vi "LP Motor Thread.vi"(11 "VISA resource name":refnum<visa-resource-name>="ASRL3::INSTR") -> ()   [LabVIEW 2015]
uses:
  MCode_LV_86/MDrive Mode.ctl
  MCode_LV_86/Set Parameter.ctl
  Stream/LP Globals.vi
  Stream/Controls/LP Motor CMD.ctl
  Stream/Controls/LP Motor Instruction.ctl
  Controls/LP Axis Enum Typedef.ctl
  Controls/LP Absolute Position Typedef.ctl
  Stream/Controls/Motor Loop Mode Typedef.ctl
  Controls/LP Motor Thread Data.ctl
  Stream/Controls/RT Streamer State.ctl
  Stream/Controls/RT Streamer Queue element.ctl
  Stream/RT Controls/RT Streamer Ack element.ctl
  MCode_LV_86/Get Parameter.ctl
  Stream/Controls/LP System State Typedef.ctl
  <vilib>/platform/TimedLoop/XDataNode/XDataNode.xnode
  <vilib>/Platform/TimedLoop/XDataNode/nitl_modes.ctl
  <vilib>/Platform/TimedLoop/XDataNode/XDNodeRunTimeDep.lvlib
  <vilib>/Platform/TimedLoop/XDataNode/wakeup.ctl
  <vilib>/Platform/TimedLoop/XDataNode/timing_clust.ctl
  Stream/Controls/LP Motor Pos And State.ctl
panel:
  out "MovedY":bool
  out "MovedR":bool
  out "MovedP":bool
  out "last error":errorcluster
  out "semaphore":T1
  out "MotorLoopMode":T2=enum."Open Loop"
  out "Working Velocity":string="10000"
  out "Hold Current":string="5"
  out "Run Current":string="50"
  out "Decel Setpoint":string="60000"
  out "Velocity":i32=10000
  out "Pitch Gain":i32=3000
  out "Roll Gain":i32=-3000
  out "RT Loop Error":errorcluster
  out "Closed Loope Cycle Time":u32
  out "open Loope Cycle Time":u32
  out "output cluster":T3
  out "MotPosition":T4
  out "CMD":T5
  out "error out":errorcluster
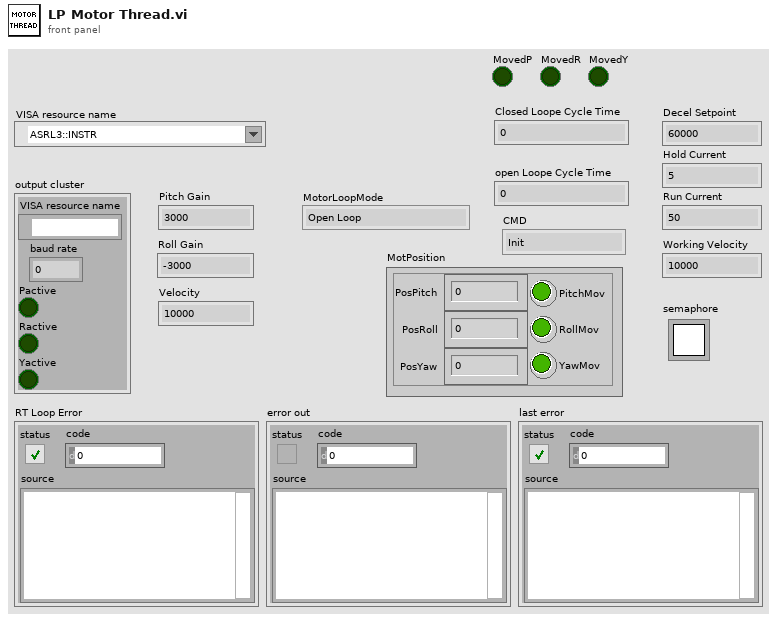
[diagram p1: front panel]
types:
  T1 = typedef "Semaphore RefNum" = refnum<k1>
  T2 = typedef "Motor Loop Mode Typedef.ctl" = enum16{"NotActive", "Open Loop", "Closed Loop", "ClosedOnce"}
  T3 = typedef "LP Motor Thread Data.ctl" = cluster{"VISA resource name":refnum<visa-resource-name>, "baud rate":u32, "Pactive":bool, "Ractive":bool, "Yactive":bool}
  T4 = typedef "LP Motor Pos And State.ctl" = cluster{"PosPitch":dbl, "PosRoll":dbl, "PosYaw":dbl, "PitchMov":bool, "RollMov":bool, "YawMov":bool}
  T5 = typedef "LP Motor CMD.ctl" = enum16{"Init", "SetAccelaration", "SetMaxVelocity", "Idle", "ClosedLoopRun", "MoveAbsolute", "MoveRelative", "MoveSRelative", "MoveSAbsolute", "StopMotors", "EnabeMotors", "SetZero", "StopMotion", "SetLoop", "FindHome", "MotorsGoToLimits", "ErrorHandling", "CloseMotor"}
  T6 = typedef "RT Streamer Ack element.ctl" = cluster{"Data":variant, "CMD":string, "error":errorcluster}
  T7 = typedef "LP System State Typedef.ctl" = cluster{"AutoLevel":bool, "MotorsEngaged":bool, "IMUok":bool}
  T8 = typedef "LP Motor Instruction.ctl" = cluster{"CMD":T5, "Data":variant}
  T9 = typedef "XDNodeRunTimeDep.lvlib/timing_clust.ctl" = cluster{"Expected End [f-1]":u64, "Actual End [f-1]":u64, "Finished Late? [f-1]":bool, "Expected End [i-1]":u64, "Actual End [i-1]":u64, "Finished Late? [i-1]":bool, "Expected Start [i]":u64, "Actual Start [i]":u64, "Expected Start [f]":u64, "Actual Start [f]":u64, "Source Name":string, "Structure Name":string, "Period":i64, "Deadline":i64, "Offset":i64, "Start":i64, "Priority":i32, "Timeout":i32, "Mode":T10, "Wakeup Reason":T11, "Error":errorcluster, "Source Type":string, "Secondary Source Type":string, "Global End Time":u64, "Global Start Time":u64, "Frame Duration":u64, "Iteration Duration":u64, "Assigned CPU":i32, "I/O Scan Engine Mode":u32}
  T10 = typedef "XDNodeRunTimeDep.lvlib/nitl_modes.ctl" = enum32{"No Change", "Process missed periods, maintain original phase", "Discard missed periods, maintain original phase", "Process missed periods, ignore original phase", "Discard missed periods, ignore original phase"}
  T11 = typedef "XDNodeRunTimeDep.lvlib/wakeup.ctl" = enum32{"Normal", "Aborted", "Asynchronous wakeup", "Timing source error", "Timed loop error", "Timeout"}
  T12 = typedef "LP Absolute Position Typedef.ctl" = cluster{"Axis":T13, "Position":dbl}
  T13 = typedef "LP Axis Enum Typedef.ctl" = enum16{"Pitch", "Roll", "Yaw"}
  T14 = typedef "Set Parameter.ctl" = enum16{"Acceleration (A)", "Baud Rate (BD)", "Counter 1 (C1)", "Counter 2 (C2)", "Control C Software Reset (CE)", "Check Sum Enable (CK)", "Clock Mode (CM)", "Clock Mode Ratio (CR)", "Clock Mode Out Step Width (CW)", "Deceleration (D)", "Digital Filtering, Input 1 (D1)", "Digital Filtering, Input 2 (D2)", "Digital Filtering, Input 3 (D3)", "Digital Filtering, Input 4 (D4)", "Digital Filtering, Input 5 (D5)", "Digital Filtering, Input 9 (D9)", "Digital Filtering, Input 10 (D10)", "Digital Filtering, Input 11 (D11)", "Digital Filtering, Input 12 (D12)", "Deadband (DB)", "Decrement Variable (DC)", "Enable/Disable Drive (DE)", "Device Name (DN)", "End Program Execution (E)", "Encoder Function Enable (EE)", "Encoder Lines (EL)", "Echo Mode (EM)", "Error Clear (ER)", "Escape (ES)", "Execute Program at Address (EX)", "Factory Default (FD)", "Hold (H)", "Hold Current (HC)", "Hold Current Encoder Index (HI)", "Home to Home Switch (HM)", "Home to Delay Time (HT)", "Increment Variable (IC)", "Initialize Parameters to NVM (IP)", "Input into Variable (IV)", "Jog Enable (JE)", "Limit Stop Mode (LM)", "Move Absolute (MA)", "Move Relative (MR)", "MicroStepping Select (MS)", "Motor Settling Delay Time (MT)", "Output 1 (O1)", "Output 2 (O2)", "Output 3 (O3)", "Output 4 (O4)", "Output 9 (O9)", "Output 10 (O10)", "Output 11 (O11)", "Output 12 (O12)", "Output High Byte (9-12) (OH)", "Output Low Byte (1-4) (OL)", "Output Total (1-4 and 9-12) (OT)", "Position (P)", "Position Maintenance (PM)", "Party Mode (PY)", "Register 1 (R1)", "Register 2 (R2)", "Register 3 (R3)", "Register 4 (R4)", "Run Current (RC)", "Stall Factor (SF)", "Slew (SL)", "Stall Mode Set (SM)", "Upgrade Firmware (UG)", "Velocity Initial (VI)", "Velocity Maximum (VM)", "Set Input #1 as Home (S1)", "Save (S)", "Save DN+PY (NameS)", "Active Party Mode (0x0A)", "Set Input #1 (S1) as Limit- Active Floating", "Set Input #2 (S2) as Limit+ Active Floating", "Set Input #1 as Home (S1) Active Floating", "Set Input #1 as Home (S2) Active Floating", "Set Input #1 (S1) as Limit+ Active Floating", "Set Input #2 (S2) as Limit- Active Floating", "Hybrid Mode (AS)"}
  T15 = typedef "RT Streamer Queue element.ctl" = cluster{"CMD":T16, "Data":variant}
  T16 = typedef "RT Streamer State.ctl" = enum16{"Init", "Idle", "Stream", "Listen", "SetRefrashRate", "SendCmdAck", "SendCmdDone", "SendSysState", "StartRecord", "Error"}
  T17 = typedef "MDrive Mode.ctl" = enum16{"Normal Mode", "Party Mode"}
  T18 = typedef "Get Parameter.ctl" = enum16{"Acceleration (A)", "Baud Rate (BD)", "Busy Flag (BY)", "Counter 1 (C1)", "Counter 2 (C2)", "Check Sum Enable (CK)", "Clock Mode (CM)", "Clock Mode Ratio (CR)", "Clock Mode Out Step Width (CW)", "Deceleration (D)", "Digital Filtering, Input 1 (D1)", "Digital Filtering, Input 2 (D2)", "Digital Filtering, Input 3 (D3)", "Digital Filtering, Input 4 (D4)", "Digital Filtering, Input 5 (D5)", "Digital Filtering, Input 9 (D9)", "Digital Filtering, Input 10 (D10)", "Digital Filtering, Input 11 (D11)", "Digital Filtering, Input 12 (D12)", "Deadband (DB)", "Enable/Disable Drive (DE)", "Device Name (DN)", "End Program Execution (E)", "Encoder Function Enable (EE)", "Encoder Lines (EL)", "Error Flag (EF)", "Error Variable (ER)", "Echo Mode (EM)", "Escape (ES)", "Execute Program at Address (EX)", "Hold Current (HC)", "Hold Current Delay Time (HI)", "Input 1 (I1)", "Input 2 (I2)", "Input 3 (I3)", "Input 4 (I4)", "Input 5 Analog (I5)", "Input 6 Encoder Index (I6)", "Input 9 (I9)", "Input 10 (I10)", "Input 11 (I11)", "Input 12 (I12)", "Input Low Byte (1-4) (IL)", "Input High Byte (9-12) (IH)", "Inputs Total (1-4,9-12) (IN)", "Internal Temperature (IT)", "Jog Enable (JE)", "Limit Stop Mode (LM)", "MicroStepping Select (MS)", "Motor Settling Delay Time (MT)", "Moving Flag (MV)", "Output 1 (O1)", "Output 2 (O2)", "Output 3 (O3)", "Output 4 (O4)", "Output 9 (O9)", "Output 10 (O10)", "Output 11 (O11)", "Output 12 (O12)", "Output High Byte (9-12) (OH)", "Output Low Byte (1-4) (OL)", "Output Total (1-4 and 9-12) (OT)", "Position (P)", "Position Captured at Trip (PC)", "Position Maintenance (PM)", "Part Number (PN)", "Party Mode (PY)", "Register 1 (R1)", "Register 2 (R2)", "Register 3 (R3)", "Register 4 (R4)", "Run Current (RC)", "Serial Number (SN)", "Stall Flag (ST)", "Stall Factor (SF)", "Stall Mode Set (SM)", "User Variables (UV)", "Velocity (V)", "Velocity Changing Flag (VC)", "Velocity Initial (VI)", "Version, Firmware (VR)", "Velocity Maximum (VM)", "Read Input1", "Read Input2"}
  T19 = cluster{dbl, i32, dbl, "MovingFlag":bool, "MovingFlag":bool, "MovingFlag":bool}
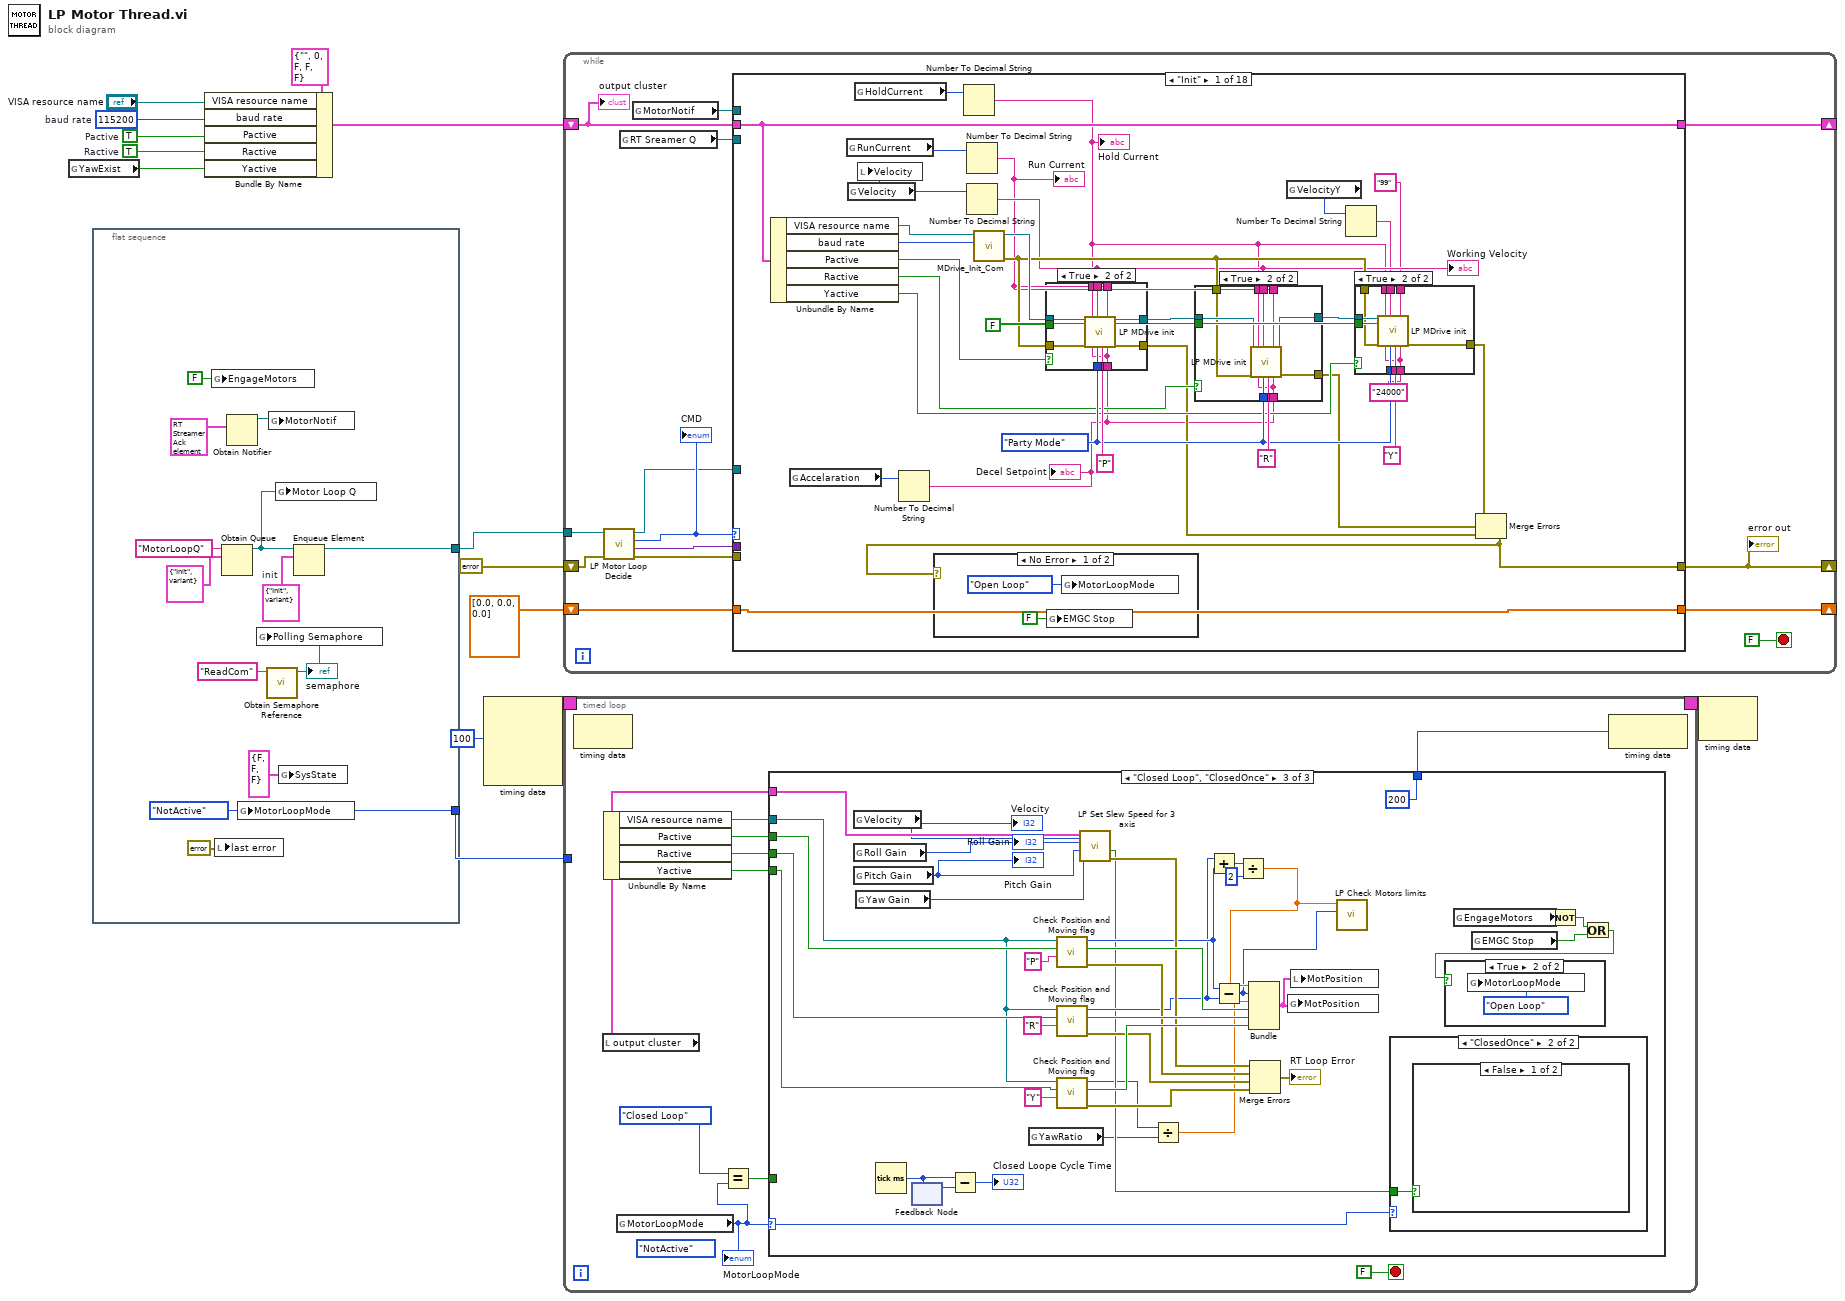
[diagram p0: block diagram]
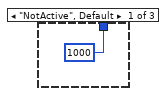
[diagram p2: hidden frame]
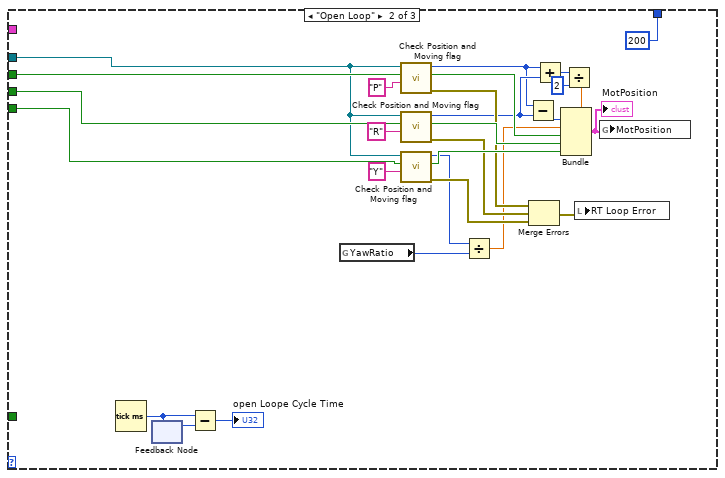
[diagram p3: hidden frame]
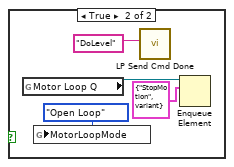
[diagram p6: hidden frame]
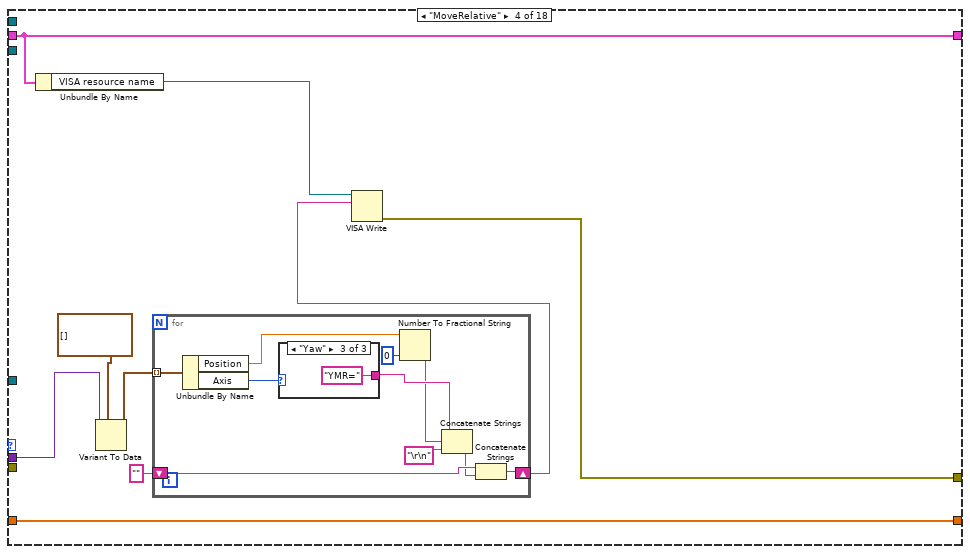
[diagram p13: hidden frame]
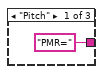
[diagram p14: hidden frame]
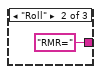
[diagram p15: hidden frame]
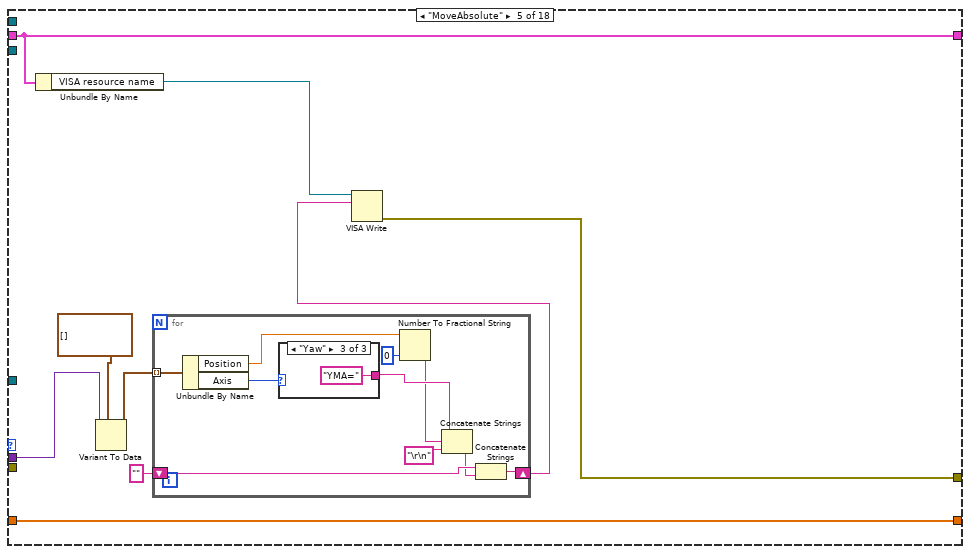
[diagram p16: hidden frame]
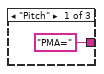
[diagram p17: hidden frame]
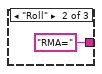
[diagram p18: hidden frame]
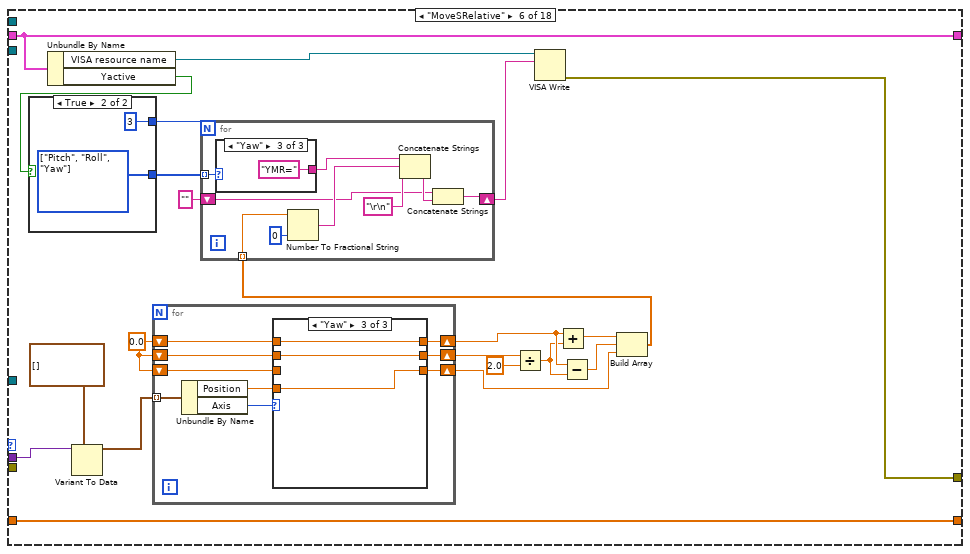
[diagram p19: hidden frame]
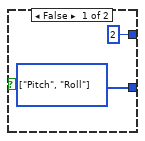
[diagram p20: hidden frame]
diagram:
  w7 = TRUE  # Ractive
  w8 = TRUE  # Pactive
  w12 = u32 115200  # baud rate
  n1 = global read "LP Globals.vi" "YawExist"() -> (w4:bool)
  n2 = flat-sequence {
    tunnel: [w23] -> w10
    tunnel: [w25] -> w9
    frame #0 {
      w22 = T8 {"CMD"=enum."Init", "Data"=variant}  # init
      w25 = Motor_Loop_Mode_Typedef."NotActive" ("MotorLoopMode")
      n3 = global write "LP Globals.vi" "EngageMotors"(FALSE ("EngageMotors")) -> ()
      n4 = local write "last error"(errorcluster {"status"=FALSE, "code"=0, "source"=""} ("last error")) -> ()
      n5 = Obtain Queue(name (unnamed)="MotorLoopQ", element data type=T8 {"CMD"=enum."Init", "Data"=variant} ("Motor Instruction")) -> (queue out=w24:refnum<queue>)  [unwired: 3 in, 2 out]
      n6 = Obtain Notifier(notification data type=T6 {"Data"=variant, "CMD"="", "error"={"status"=FALSE, "code"=0, "source"=""}} ("Cluster")) -> (notifier out=w16:refnum<notifier>)  [unwired: 3 in, 2 out]
      n7 = global write "LP Globals.vi" "MotorLoopMode"(w25) -> ()
      n8 = call <vilib>:"Obtain Semaphore Reference.vi"("name (unnamed)"="ReadCom") -> ("semaphore"=w20:T1)  [unwired: 4 in, 2 out]
      "semaphore" <- w20
      n9 = global write "LP Globals.vi" "Polling Semaphore"(w20) -> ()
      n10 = global write "LP Globals.vi" "MotorNotif"(w16) -> ()
      n11 = global write "LP Globals.vi" "Motor Loop Q"(w24) -> ()
      n12 = global write "LP Globals.vi" "SysState"(T7 {"AutoLevel"=FALSE, "MotorsEngaged"=FALSE, "IMUok"=FALSE} ("SysState")) -> ()
      n13 = Enqueue Element(queue=w24, element=w22) -> (queue out=w23:refnum<queue>)  [unwired: 2 in, 2 out]
    }
  }
  n14 = Bundle By Name(cluster=T3 {"VISA resource name"="", "baud rate"=0, "Pactive"=FALSE, "Ractive"=FALSE, "Yactive"=FALSE} ("output cluster"), "VISA resource name"="VISA resource name", "baud rate"=w12, "Pactive"=w8, "Ractive"=w7, "Yactive"=w4) -> (w11:T3)
  n15 = node-c288(i64 100 ("Period")) -> (w3:T9)  [unwired: 3 in]
  n16 = while {
    tunnel: w10 -> [w40]
    shift-right: [w36] -> _
    shift-left: errorcluster {"status"=FALSE, "code"=0, "source"=""} ("error out") -> [w38]
    shift-right: [w37] -> _
    shift-left: w11 -> [w32]
    shift-right: [w30] -> _
    shift-left: dbl[] [0.0, 0.0, 0.0] -> [w31]
    stop <- FALSE stop-if-true
    n17 = call "LP Motor Loop Decide.vi"("error in (no error)"=w38, "Queue in"=w40) -> ("error out"=w39:errorcluster, "Data"=w35:variant, "CMD"=w34:T5, "queue out"=w33:refnum<queue>)  [unwired: 6 in]
    "CMD" <- w34
    n18 = global read "LP Globals.vi" "RT Sreamer Q"() -> (w29:refnum<queue>)
    n19 = global read "LP Globals.vi" "MotorNotif"() -> (w28:refnum<notifier>)
    n20 = case shown="\"Init\"" w34 {
      tunnel: w35 -> [_ _ _ w124 w146 w180 _ w238 w292 w307 _ w362 _ w462 _ _ _ _]
      tunnel: w39 -> [_ w113 w114 _ _ _ _ _ _ _ _ _ _ _ _ _ w535 w540]
      tunnel: [w55 w113 w114 w118 w140 w176 w217 w234 w286 w305 w328 w350 w427 w461 w476 w507 _ w540] -> w36
      tunnel: w32 -> [w71 w112 w116 w125 w147 w181 w218 w239 w294 w309 w334 w371 w443 w466 w482 w511 w536 w539]
      tunnel: [w71 w112 w116 w125 w147 w181 w218 w239 w294 w309 w334 w371 w443 w466 w482 w511 w536 w539] -> w37
      tunnel: w33 -> [_ _ _ _ _ _ _ _ _ _ _ _ _ w460 _ _ _ _]
      tunnel: w31 -> [w54 w111 w115 w117 w139 w164 w216 w225 w281 w302 w323 w361 w433 w459 w471 w499 w533 w537]
      tunnel: [w54 w111 w115 w117 w139 w164 w216 w224 w281 w302 w323 w361 w433 w459 w471 w499 w533 w537] -> w30
      tunnel: w29 -> [_ _ _ _ _ _ _ _ _ _ _ _ w432 _ _ _ _ _]
      tunnel: w28 -> [_ _ _ _ _ _ _ _ _ _ _ _ w426 _ _ _ _ _]
      frame "Init" {
        w63 = FALSE ("Factory Default")
        w65 = MDrive_Mode."Party Mode" ("Mdrive Mode")
        n21 = Unbundle By Name(w71) -> ("VISA resource name"=w73:refnum<visa-resource-name>, "baud rate"=w72:u32, "Pactive"=w62:bool, "Ractive"=w61:bool, "Yactive"=w60:bool)
        n22 = global read "LP Globals.vi" "Accelaration"() -> (w52:i32)
        n23 = global read "LP Globals.vi" "RunCurrent"() -> (w48:i32)
        n24 = global read "LP Globals.vi" "Velocity"() -> (w46:i32)
        n25 = global read "LP Globals.vi" "HoldCurrent"() -> (w50:i32)
        n26 = local write "Velocity"(w46) -> ()
        n27 = Number To Decimal String(number=w52) -> (decimal integer string=w51:string)  [unwired: 1 in]
        "Decel Setpoint" <- w51
        n28 = Number To Decimal String(number=w50) -> (decimal integer string=w49:string)  [unwired: 1 in]
        "Hold Current" <- w49
        n29 = Number To Decimal String(number=w48) -> (decimal integer string=w47:string)  [unwired: 1 in]
        "Run Current" <- w47
        n30 = Number To Decimal String(number=w46) -> (decimal integer string=w53:string)  [unwired: 1 in]
        "Working Velocity" <- w53
        n31 = call "MDrive_Init_Com.vi"("baud rate"=w72, "VISA resource name"=w73) -> ("error out"=w56:errorcluster, "VISA resource name out"=w70:refnum<visa-resource-name>)  [unwired: 8 in]
        n32 = case shown="True" w62 {
          tunnel: w70 -> [w97 w108]
          tunnel: [w97 w107] -> w69
          tunnel: [w96 w99] -> w57
          tunnel: "P" ("Device Name") -> [_ w106]
          tunnel: w65 -> [_ w105]
          tunnel: w51 -> [_ w104]
          tunnel: w47 -> [_ w103]
          tunnel: w49 -> [_ w102]
          tunnel: w53 -> [_ w101]
          tunnel: w63 -> [_ w100]
          tunnel: w56 -> [w96 w98]
          frame False {
          }
          frame True {
            n33 = call "LP MDrive init.vi"("VISA IN"=w108, "Factory Default"=w100, "error in"=w98, "Hold Current"=w102, "Accel Setpoint"=w104, "Working Velocity"=w101, "Mdrive Mode"=w105, "Device Name"=w106, "Run Current"=w103, "Decel Setpoint"=w104) -> ("VISA OUT"=w107:refnum<visa-resource-name>, "error out"=w99:errorcluster)  [unwired: 8 in]
          }
        }
        n34 = case shown="True" w61 {
          tunnel: w69 -> [w84 w95]
          tunnel: "R" ("Device Name") -> [_ w94]
          tunnel: [_ w93] -> w58
          tunnel: [w84 w92] -> w66
          tunnel: w65 -> [_ w91]
          tunnel: w51 -> [_ w90]
          tunnel: w47 -> [_ w89]
          tunnel: w49 -> [_ w88]
          tunnel: w53 -> [_ w87]
          tunnel: w63 -> [_ w86]
          tunnel: w56 -> [_ w85]
          frame False {
          }
          frame True {
            n35 = call "LP MDrive init.vi"("VISA IN"=w95, "Factory Default"=w86, "error in"=w85, "Hold Current"=w88, "Accel Setpoint"=w90, "Working Velocity"=w87, "Mdrive Mode"=w91, "Device Name"=w94, "Run Current"=w89, "Decel Setpoint"=w90) -> ("VISA OUT"=w92:refnum<visa-resource-name>, "error out"=w93:errorcluster)  [unwired: 8 in]
          }
        }
        n36 = global read "LP Globals.vi" "VelocityY"() -> (w43:i32)
        n37 = Number To Decimal String(number=w43) -> (decimal integer string=w45:string)  [unwired: 1 in]
        n38 = case shown="True" w60 {
          tunnel: w66 -> [_ w83]
          tunnel: w65 -> [_ w82]
          tunnel: "Y" ("Device Name") -> [_ w81]
          tunnel: "24000" -> [_ w80]
          tunnel: "99" ("decimal integer string") -> [_ w79]
          tunnel: w49 -> [_ w78]
          tunnel: [_ w77] -> w59
          tunnel: w63 -> [_ w76]
          tunnel: w56 -> [_ w75]
          tunnel: w45 -> [_ w74]
          frame False {
          }
          frame True {
            n39 = call "LP MDrive init.vi"("VISA IN"=w83, "Factory Default"=w76, "error in"=w75, "Hold Current"=w78, "Accel Setpoint"=w80, "Working Velocity"=w74, "Mdrive Mode"=w82, "Device Name"=w81, "Run Current"=w79, "Decel Setpoint"=w80) -> ("error out"=w77:errorcluster)  [unwired: 8 in, 1 out]
          }
        }
        n40 = Merge Errors(w59, w58, w57) -> (w55:errorcluster)
        n41 = case shown="No Error" w55 {
          frame No Error {
            n42 = global write "LP Globals.vi" "EMGC Stop"(FALSE ("EMGC Stop")) -> ()
            n43 = global write "LP Globals.vi" "MotorLoopMode"(Motor_Loop_Mode_Typedef."Open Loop" ("MotorLoopMode")) -> ()
          }
          frame Error {
          }
        }
      }
      frame "Idle" {
      }
      frame "ClosedLoopRun" {
      }
      frame "MoveRelative" {
        n44 = Unbundle By Name(w125) -> ("VISA resource name"=w119:refnum<visa-resource-name>)
        n45 = Variant To Data(type=T12[] [], Variant=w124) -> (data=w123:T12[])  [unwired: 1 in, 1 out]
        n46 = for {
          tunnel: w123 -> [w135] mode=indexing
          shift-right: [w126] -> w120
          shift-left: "" -> [w128]
          n47 = Unbundle By Name(w135) -> ("Position"=w133:dbl, "Axis"=w134:T13)
          n48 = case shown="\"Yaw\"" w134 {
            tunnel: ["PMR=" "RMR=" "YMR="] -> w131
            frame "Pitch" {
            }
            frame "Roll" {
            }
            frame "Yaw" {
            }
          }
          n49 = Number To Fractional String(number=w133, precision (6)=i16 0) -> (F-format string=w130:string)  [unwired: 2 in]
          n50 = Concatenate Strings(w131, w130, "\r\n") -> (w127:string)
          n51 = Concatenate Strings(w128, w127) -> (w126:string)
        }
        n52 = VISA Write(VISA resource name=w119, write buffer=w120) -> (error out=w118:errorcluster)  [unwired: 1 in, 2 out]
      }
      frame "MoveAbsolute" {
        n53 = Unbundle By Name(w147) -> ("VISA resource name"=w141:refnum<visa-resource-name>)
        n54 = Variant To Data(type=T12[] [], Variant=w146) -> (data=w145:T12[])  [unwired: 1 in, 1 out]
        n55 = for {
          tunnel: w145 -> [w157] mode=indexing
          shift-right: [w148] -> w142
          shift-left: "" -> [w150]
          n56 = Unbundle By Name(w157) -> ("Position"=w155:dbl, "Axis"=w156:T13)
          n57 = case shown="\"Yaw\"" w156 {
            tunnel: ["PMA=" "RMA=" "YMA="] -> w153
            frame "Pitch" {
            }
            frame "Roll" {
            }
            frame "Yaw" {
            }
          }
          n58 = Number To Fractional String(number=w155, precision (6)=i16 0) -> (F-format string=w152:string)  [unwired: 2 in]
          n59 = Concatenate Strings(w153, w152, "\r\n") -> (w149:string)
          n60 = Concatenate Strings(w150, w149) -> (w148:string)
        }
        n61 = VISA Write(VISA resource name=w141, write buffer=w142) -> (error out=w140:errorcluster)  [unwired: 1 in, 2 out]
      }
      frame "MoveSRelative" {
        w175 = 0.0 ("Position")
        n62 = Unbundle By Name(w181) -> ("VISA resource name"=w177:refnum<visa-resource-name>, "Yactive"=w161:bool)
        n63 = case shown="True" w161 {
          tunnel: [w183 w185] -> w169
          tunnel: [2 3] -> w162
          frame False {
            w183 = T13[] [enum."Pitch", enum."Roll"] items=["Pitch", "Roll", "Yaw"]
          }
          frame True {
            w185 = T13[] [enum."Pitch", enum."Roll", enum."Yaw"] items=["Pitch", "Roll", "Yaw"]
          }
        }
        n64 = Variant To Data(type=T12[] [], Variant=w180) -> (data=w179:T12[])  [unwired: 1 in, 1 out]
        n65 = for {
          tunnel: w179 -> [w206] mode=indexing
          shift-right: [w202] -> w174
          shift-left: w175 -> [w200]
          shift-right: [w204] -> w172
          shift-left: w175 -> [w198]
          shift-right: [w201] -> w163
          shift-left: w175 -> [w199]
          n66 = Unbundle By Name(w206) -> ("Position"=w203:dbl, "Axis"=w205:T13)
          n67 = case shown="\"Yaw\"" w205 {
            tunnel: [w207 w212 w215] -> w204
            tunnel: w203 -> [w207 w210 w213]
            tunnel: [w209 w210 w214] -> w202
            tunnel: [w208 w211 w213] -> w201
            tunnel: w200 -> [w209 _ w214]
            tunnel: w199 -> [w208 w211 _]
            tunnel: w198 -> [_ w212 w215]
            frame "Pitch" {
            }
            frame "Roll" {
            }
            frame "Yaw" {
            }
          }
        }
        n68 = Divide(x=w174, y=2.0) -> (x/y=w171:dbl)
        n69 = Add(x=w172, y=w171) -> (x+y=w168:dbl)
        n70 = Subtract(x=w172, y=w171) -> (x-y=w167:dbl)
        n71 = Build Array(w168, w167, w163) -> (w166:dbl[])
        n72 = for {
          N: w162 -> [_]
          shift-right: [w189] -> w165
          shift-left: "" -> [w188]
          tunnel: w169 -> [w187] mode=indexing
          tunnel: w166 -> [w186] mode=indexing
          n73 = case shown="\"Yaw\"" w187 {
            tunnel: ["PMR=" "RMR=" "YMR="] -> w190
            frame "Pitch" {
            }
            frame "Roll" {
            }
            frame "Yaw" {
            }
          }
          n74 = Number To Fractional String(number=w186, precision (6)=i16 0) -> (F-format string=w192:string)  [unwired: 2 in]
          n75 = Concatenate Strings(w190, w192, "\r\n") -> (w194:string)
          n76 = Concatenate Strings(w188, w194) -> (w189:string)
        }
        n77 = VISA Write(VISA resource name=w177, write buffer=w165) -> (error out=w176:errorcluster)  [unwired: 1 in, 2 out]
      }
      frame "MotorsGoToLimits" {
        n78 = call "MotorsGoToLimits.vi"("output cluster"=w218) -> ("error out"=w217:errorcluster)  [unwired: 10 in]
      }
      frame "MoveSAbsolute" {
        n79 = Unbundle By Name(w239) -> ("VISA resource name"=w235:refnum<visa-resource-name>, "Yactive"=w221:bool)
        n80 = case shown="True" w221 {
          tunnel: [w241 w243] -> w230
          tunnel: [2 3] -> w219
          frame False {
            w241 = T13[] [enum."Pitch", enum."Roll"] items=["Pitch", "Roll", "Yaw"]
          }
          frame True {
            w243 = T13[] [enum."Pitch", enum."Roll", enum."Yaw"] items=["Pitch", "Roll", "Yaw"]
          }
        }
        n81 = Variant To Data(type=T12[] [], Variant=w238) -> (data=w237:T12[])  [unwired: 1 in, 1 out]
        n82 = for {
          tunnel: w237 -> [w260] mode=indexing
          shift-right: [w256] -> w224
          shift-left: w225 -> [w257]
          n83 = Unbundle By Name(w260) -> ("Position"=w258:dbl, "Axis"=w259:T13)
          n84 = case shown="\"Pitch\"" w259 {
            tunnel: w258 -> [w262 w268 w274]
            tunnel: w257 -> [w266 w272 w278]
            tunnel: [w264 w270 w276] -> w256
            frame "Pitch" {
              n85 = global read "LP Globals.vi" "PitchRatio"() -> (w263:i32)
              n86 = Multiply(x=w263, y=w262) -> (x*y=w261:dbl)
              n87 = Replace Array Subset(array=w266, new element=w261, index=0) -> (w264:dbl[])
            }
            frame "Roll" {
              n88 = global read "LP Globals.vi" "RollRatio"() -> (w269:i32)
              n89 = Multiply(x=w269, y=w268) -> (x*y=w267:dbl)
              n90 = Replace Array Subset(array=w272, new element=w267, index=1) -> (w270:dbl[])
            }
            frame "Yaw" {
              n91 = global read "LP Globals.vi" "YawRatio"() -> (w273:i32)
              n92 = Multiply(x=w273, y=w274) -> (x*y=w275:dbl)
              n93 = Replace Array Subset(array=w278, new element=w275, index=2) -> (w276:dbl[])
            }
          }
        }
        n94 = Index Array(array=w224) -> (element #1=w223:dbl, element #2=w222:dbl, element #3=w220:dbl)  [unwired: 3 in]
        n95 = Divide(x=w222, y=2.0) -> (x/y=w232:dbl)
        n96 = Add(x=w223, y=w232) -> (x+y=w229:dbl)
        n97 = Subtract(x=w223, y=w232) -> (x-y=w228:dbl)
        n98 = Build Array(w229, w228, w220) -> (w227:dbl[])
        n99 = for {
          N: w219 -> [_]
          shift-right: [w247] -> w226
          shift-left: "" -> [w246]
          tunnel: w230 -> [w245] mode=indexing
          tunnel: w227 -> [w244] mode=indexing
          n100 = case shown="\"Yaw\"" w245 {
            tunnel: ["PMA=" "RMA=" "YMA="] -> w248
            frame "Pitch" {
            }
            frame "Roll" {
            }
            frame "Yaw" {
            }
          }
          n101 = Number To Fractional String(number=w244, precision (6)=i16 0) -> (F-format string=w250:string)  [unwired: 2 in]
          n102 = Concatenate Strings(w248, w250, "\r\n") -> (w252:string)
          n103 = Concatenate Strings(w246, w252) -> (w247:string)
        }
        n104 = VISA Write(VISA resource name=w235, write buffer=w226) -> (error out=w234:errorcluster)  [unwired: 1 in, 2 out]
      }
      frame "SetAccelaration" {
        n105 = Variant To Data(type=T12 {"Axis"=enum."Roll", "Position"=0.0} ("AbsolutePosition"), Variant=w292) -> (data=w290:T12)  [unwired: 1 in, 1 out]
        n106 = Unbundle By Name(w294) -> ("VISA resource name"=w293:refnum<visa-resource-name>)
        n107 = Unbundle By Name(w290) -> ("Position"=w288:dbl, "Axis"=w289:T13)
        n108 = Number To Fractional String(number=w288, precision (6)=i16 0) -> (F-format string=w280:string)  [unwired: 2 in]
        n109 = case shown="\"Yaw\"" w289 {
          tunnel: ["P" "R" "Y"] -> w283
          tunnel: [w296 w298 "24000"] -> w279
          tunnel: w280 -> [w296 w298 _]
          frame "Pitch" {
          }
          frame "Roll" {
          }
          frame "Yaw" {
          }
        }
        n110 = call "MDrive_Set_Parameter.vi"("Device Name"=w283, "Parameter Setpoint"=w279, "Set Parameter"=Set_Parameter."Acceleration (A)", "VISA IN"=w293) -> ("error out"=w287:errorcluster, "VISA OUT"=w285:refnum<visa-resource-name>)  [unwired: 5 in, 1 out]
        n111 = call "MDrive_Set_Parameter.vi"("Device Name"=w283, "error in"=w287, "Parameter Setpoint"=w279, "Set Parameter"=Set_Parameter."Deceleration (D)", "VISA IN"=w285) -> ("error out"=w286:errorcluster)  [unwired: 4 in, 2 out]
      }
      frame "SetMaxVelocity" {
        n112 = Variant To Data(type=T12[] [], Variant=w307) -> (data=w306:T12[])  [unwired: 1 in, 1 out]
        n113 = Unbundle By Name(w309) -> ("VISA resource name"=w308:refnum<visa-resource-name>)
        n114 = for {
          tunnel: w308 -> [w318]
          tunnel: w306 -> [w317] mode=indexing
          shift-right: [w312] -> w305
          shift-left: errorcluster {"status"=FALSE, "code"=0, "source"=""} ("error out") -> [w311]
          n115 = Unbundle By Name(w317) -> ("Position"=w315:dbl, "Axis"=w316:T13)
          n116 = case shown="\"Pitch\"" w316 {
            tunnel: ["P" "R" "Y"] -> w313
            frame "Pitch" {
            }
            frame "Roll" {
            }
            frame "Yaw" {
            }
          }
          n117 = Number To Fractional String(number=w315, precision (6)=i16 0) -> (F-format string=w314:string)  [unwired: 2 in]
          n118 = call "MDrive_Set_Parameter.vi"("Device Name"=w313, "error in"=w311, "Parameter Setpoint"=w314, "Set Parameter"=Set_Parameter."Velocity Maximum (VM)", "VISA IN"=w318) -> ("error out"=w312:errorcluster)  [unwired: 4 in, 2 out]
        }
      }
      frame "StopMotors" {
        (unwired) "0" ("Parameter Setpoint")
        w332 = "\u001b" ("Parameter Setpoint")
        w327 = Set_Parameter."Enable/Disable Drive (DE)" ("Set Parameter")
        n119 = Unbundle By Name(w334) -> ("VISA resource name"=w333:refnum<visa-resource-name>, "Pactive"=w324:bool, "Ractive"=w325:bool, "Yactive"=w326:bool)
        n120 = case shown="True" w326 {
          tunnel: w333 -> [_ w339]
          tunnel: w327 -> [_ w338]
          tunnel: w332 -> [_ w336]
          tunnel: [_ w335] -> w329
          frame False {
          }
          frame True {
            n121 = call "MDrive_Set_Parameter.vi"("Device Name"="Y", "Parameter Setpoint"=w336, "Set Parameter"=w338, "VISA IN"=w339) -> ("error out"=w335:errorcluster)  [unwired: 5 in, 2 out]
          }
        }
        n122 = case shown="True" w325 {
          tunnel: w333 -> [_ w344]
          tunnel: w327 -> [_ w343]
          tunnel: w332 -> [_ w341]
          tunnel: [_ w340] -> w330
          frame False {
          }
          frame True {
            n123 = call "MDrive_Set_Parameter.vi"("Device Name"="R", "Parameter Setpoint"=w341, "Set Parameter"=w343, "VISA IN"=w344) -> ("error out"=w340:errorcluster)  [unwired: 5 in, 2 out]
          }
        }
        n124 = case shown="True" w324 {
          tunnel: w333 -> [_ w349]
          tunnel: w327 -> [_ w348]
          tunnel: w332 -> [_ w346]
          tunnel: [_ w345] -> w331
          frame False {
          }
          frame True {
            n125 = call "MDrive_Set_Parameter.vi"("Device Name"="P", "Parameter Setpoint"=w346, "Set Parameter"=w348, "VISA IN"=w349) -> ("error out"=w345:errorcluster)  [unwired: 5 in, 2 out]
          }
        }
        n126 = Merge Errors(w331, w330, w329) -> (w328:errorcluster)
      }
      frame "EnabeMotors" {
        w359 = u16 2000 ("Timeout")
        w360 = Get_Parameter."Enable/Disable Drive (DE)" ("Get Parameter")
        w369 = Set_Parameter."Enable/Disable Drive (DE)" ("Set Parameter")
        n127 = Unbundle By Name(w371) -> ("VISA resource name"=w370:refnum<visa-resource-name>, "Pactive"=w366:bool, "Ractive"=w365:bool, "Yactive"=w364:bool)
        n128 = Variant To Data(type=TRUE, Variant=w362) -> (data=w351:bool)  [unwired: 1 in, 1 out]
        n129 = case shown="False" w351 {
          tunnel: ["0" ("Parameter Setpoint") "1" ("Parameter Setpoint")] -> w358
          frame False {
          }
          frame True {
          }
        }
        n130 = Decimal String To Number(string=w358) -> (number=w357:i32)  [unwired: 2 in, 1 out]
        n131 = case shown="True" w364 {
          tunnel: w370 -> [_ w404]
          tunnel: w369 -> [_ w403]
          tunnel: w358 -> [_ w402]
          tunnel: [_ w400] -> w367
          tunnel: w360 -> [_ w397]
          tunnel: w359 -> [_ w396]
          tunnel: w357 -> [_ w395]
          frame False {
          }
          frame True {
            w399 = "Y" ("Device Name")
            n132 = call "MDrive_Set_Parameter.vi"("Device Name"=w399, "Parameter Setpoint"=w402, "Set Parameter"=w403, "VISA IN"=w404) -> ("error out"=w401:errorcluster, "VISA OUT"=w398:refnum<visa-resource-name>)  [unwired: 5 in, 1 out]
            n133 = call "Wait For CMD Ack.vi"("Timeout"=w396, "Device Name"=w399, "error in (no error)"=w401, "Get Parameter"=w397, "ExpectedValue"=w395, "VISA Refnum in"=w398) -> ("error out"=w400:errorcluster)  [unwired: 4 in, 1 out]
          }
        }
        n134 = case shown="True" w366 {
          tunnel: w370 -> [_ w424]
          tunnel: w369 -> [_ w423]
          tunnel: w358 -> [_ w422]
          tunnel: [_ w419] -> w356
          tunnel: w360 -> [_ w421]
          tunnel: w359 -> [_ w416]
          tunnel: w357 -> [_ w415]
          frame False {
          }
          frame True {
            w417 = "P" ("Device Name")
            n135 = call "MDrive_Set_Parameter.vi"("Device Name"=w417, "Parameter Setpoint"=w422, "Set Parameter"=w423, "VISA IN"=w424) -> ("error out"=w420:errorcluster, "VISA OUT"=w418:refnum<visa-resource-name>)  [unwired: 5 in, 1 out]
            n136 = call "Wait For CMD Ack.vi"("Timeout"=w416, "Device Name"=w417, "error in (no error)"=w420, "Get Parameter"=w421, "ExpectedValue"=w415, "VISA Refnum in"=w418) -> ("error out"=w419:errorcluster)  [unwired: 4 in, 1 out]
          }
        }
        n137 = case shown="True" w365 {
          tunnel: w370 -> [_ w414]
          tunnel: w369 -> [_ w413]
          tunnel: w358 -> [_ w412]
          tunnel: [_ w410] -> w368
          tunnel: w360 -> [_ w408]
          tunnel: w359 -> [_ w406]
          tunnel: w357 -> [_ w405]
          frame False {
          }
          frame True {
            w409 = "R" ("Device Name")
            n138 = call "MDrive_Set_Parameter.vi"("Device Name"=w409, "Parameter Setpoint"=w412, "Set Parameter"=w413, "VISA IN"=w414) -> ("error out"=w411:errorcluster, "VISA OUT"=w407:refnum<visa-resource-name>)  [unwired: 5 in, 1 out]
            n139 = call "Wait For CMD Ack.vi"("Timeout"=w406, "Device Name"=w409, "error in (no error)"=w411, "Get Parameter"=w408, "ExpectedValue"=w405, "VISA Refnum in"=w407) -> ("error out"=w410:errorcluster)  [unwired: 4 in, 1 out]
          }
        }
        n140 = Merge Errors(w356, w368, w367) -> (w350:errorcluster)
        n141 = case shown="False" w351 {
          tunnel: w350 -> [w388 w391]
          tunnel: [w387 w390] -> w355
          frame False {
            n142 = case shown="No Error" w388 {
              tunnel: [_ w389] -> w387
              frame No Error {
              }
              frame Error {
                n143 = global read "LP Globals.vi" "EngageMotors"() -> (w389:bool)
              }
            }
          }
          frame True {
            n144 = case shown="No Error" w391 {
              tunnel: [TRUE ("EngageMotors") _] -> w390
              frame No Error {
              }
              frame Error {
              }
            }
          }
        }
        n145 = global write "LP Globals.vi" "EngageMotors"(w355) -> ()
        n146 = feedback #1(u8 0) -> (w352:u8)
        n147 = case shown="Error" w350 {
          selector: w350 -> [w372 w376]
          tunnel: [u8 0 w377] -> w353
          tunnel: w352 -> [_ w378]
          tunnel: w351 -> [_ w375]
          frame No Error {
            n148 = call "LP Send Cmd Done.vi"("error in (no error)"=w372, "CMD"="EngageMotor") -> ()  [unwired: 10 in]
          }
          frame Error {
            n149 = case shown="0..3" w378 {
              selector: w378 -> [_ w386]
              tunnel: [_ w385] -> w377
              tunnel: w376 -> [w379 _]
              tunnel: w375 -> [_ w381]
              frame Default {
                n150 = call "LP Send Cmd Done.vi"("error in (no error)"=w379, "CMD"="EngageMotor") -> ()  [unwired: 10 in]
              }
              frame 0..3 {
                n151 = global read "LP Globals.vi" "Motor Loop Q"() -> (w384:refnum<queue>)
                n152 = Increment(x=w386) -> (x+1=w385:u8)
                n153 = Bundle By Name(cluster=T8 {"CMD"=enum."EnabeMotors", "Data"=variant} ("element"), "Data"=w381) -> (w382:T8)
                n154 = Enqueue Element(queue=w384, element=w382) -> ()  [unwired: 2 in, 3 out]
              }
            }
          }
        }
        n155 = feedback-in #1(w353) -> ()
      }
      frame "SetZero" {
        w434 = "0" ("Parameter Setpoint")
        w441 = Set_Parameter."Position (P)" ("Set Parameter")
        n156 = Unbundle By Name(w443) -> ("VISA resource name"=w442:refnum<visa-resource-name>, "Pactive"=w437:bool, "Ractive"=w436:bool, "Yactive"=w435:bool)
        n157 = case shown="True" w435 {
          tunnel: w442 -> [_ w448]
          tunnel: w441 -> [_ w447]
          tunnel: w434 -> [_ w445]
          tunnel: [_ w444] -> w438
          frame False {
          }
          frame True {
            n158 = call "MDrive_Set_Parameter.vi"("Device Name"="Y", "Parameter Setpoint"=w445, "Set Parameter"=w447, "VISA IN"=w448) -> ("error out"=w444:errorcluster)  [unwired: 5 in, 2 out]
          }
        }
        n159 = case shown="True" w437 {
          tunnel: w442 -> [_ w458]
          tunnel: w441 -> [_ w457]
          tunnel: w434 -> [_ w455]
          tunnel: [_ w454] -> w440
          frame False {
          }
          frame True {
            n160 = call "MDrive_Set_Parameter.vi"("Device Name"="P", "Parameter Setpoint"=w455, "Set Parameter"=w457, "VISA IN"=w458) -> ("error out"=w454:errorcluster)  [unwired: 5 in, 2 out]
          }
        }
        n161 = case shown="True" w436 {
          tunnel: w442 -> [_ w453]
          tunnel: w441 -> [_ w452]
          tunnel: w434 -> [_ w450]
          tunnel: [_ w449] -> w439
          frame False {
          }
          frame True {
            n162 = call "MDrive_Set_Parameter.vi"("Device Name"="R", "Parameter Setpoint"=w450, "Set Parameter"=w452, "VISA IN"=w453) -> ("error out"=w449:errorcluster)  [unwired: 5 in, 2 out]
          }
        }
        n163 = Merge Errors(w440, w439, w438) -> (w427:errorcluster)
        n164 = Bundle By Name(cluster=T6 {"Data"=variant, "CMD"="", "error"={"status"=FALSE, "code"=0, "source"=""}} ("Cluster"), "CMD"="AxisZero", "error"=w427) -> (w425:T6)
        n165 = Bundle By Name(cluster=T15 {"CMD"=enum."SendCmdDone", "Data"=variant} ("element"), "Data"=w425) -> (w430:T15)
        n166 = Send Notification(notification=w425, notifier=w426) -> ()  [unwired: 1 in, 2 out]
        n167 = Enqueue Element(queue=w432, element=w430) -> ()  [unwired: 2 in, 3 out]
      }
      frame "SetLoop" {
        n168 = Variant To Data(type=FALSE, Variant=w462) -> (data=w464:bool, error out=w461:errorcluster)  [unwired: 1 in]
        n169 = case shown="False" w464 {
          tunnel: [Motor_Loop_Mode_Typedef."Open Loop" ("MotorLoopMode") Motor_Loop_Mode_Typedef."Closed Loop" ("MotorLoopMode")] -> w463
          tunnel: w460 -> [w468 _]
          frame False {
            n170 = Enqueue Element(queue=w468, element=T8 {"CMD"=enum."StopMotion", "Data"=variant}) -> ()  [unwired: 2 in, 3 out]
          }
          frame True {
          }
        }
        n171 = global write "LP Globals.vi" "MotorLoopMode"(w463) -> ()
      }
      frame "StopMotion" {
        w472 = "1" ("Parameter Setpoint")
        w480 = Set_Parameter."Move Relative (MR)" ("Set Parameter")
        n172 = Unbundle By Name(w482) -> ("VISA resource name"=w481:refnum<visa-resource-name>, "Pactive"=w475:bool, "Ractive"=w474:bool, "Yactive"=w473:bool)
        n173 = case shown="True" w473 {
          tunnel: w481 -> [_ w487]
          tunnel: w480 -> [_ w486]
          tunnel: w472 -> [_ w484]
          tunnel: [_ w483] -> w477
          frame False {
          }
          frame True {
            n174 = call "MDrive_Set_Parameter.vi"("Device Name"="Y", "Parameter Setpoint"=w484, "Set Parameter"=w486, "VISA IN"=w487) -> ("error out"=w483:errorcluster)  [unwired: 5 in, 2 out]
          }
        }
        n175 = case shown="True" w475 {
          tunnel: w481 -> [_ w497]
          tunnel: w480 -> [_ w496]
          tunnel: w472 -> [_ w494]
          tunnel: [_ w493] -> w479
          frame False {
          }
          frame True {
            n176 = call "MDrive_Set_Parameter.vi"("Device Name"="P", "Parameter Setpoint"=w494, "Set Parameter"=w496, "VISA IN"=w497) -> ("error out"=w493:errorcluster)  [unwired: 5 in, 2 out]
          }
        }
        n177 = case shown="True" w474 {
          tunnel: w481 -> [_ w492]
          tunnel: w480 -> [_ w491]
          tunnel: w472 -> [_ w489]
          tunnel: [_ w488] -> w478
          frame False {
          }
          frame True {
            n178 = call "MDrive_Set_Parameter.vi"("Device Name"="R", "Parameter Setpoint"=w489, "Set Parameter"=w491, "VISA IN"=w492) -> ("error out"=w488:errorcluster)  [unwired: 5 in, 2 out]
          }
        }
        n179 = Merge Errors(w479, w478, w477) -> (w476:errorcluster)
      }
      frame "FindHome" {
        w500 = "5000" ("Max Velocity to Home")
        w501 = MDrive_Mode."Party Mode" ("Mdrive Mode")
        w502 = "1" ("Home Direction")
        n180 = Unbundle By Name(w511) -> ("VISA resource name"=w503:refnum<visa-resource-name>, "Pactive"=w510:bool, "Ractive"=w509:bool, "Yactive"=w508:bool)
        n181 = case shown="True" w510 {
          tunnel: w503 -> [_ w532]
          tunnel: [_ w531] -> w506
          tunnel: w502 -> [_ w529]
          tunnel: w501 -> [_ w528]
          tunnel: w500 -> [_ w527]
          frame False {
          }
          frame True {
            n182 = call "LP MDrive_Home.vi"("VISA IN"=w532, "Home Direction"=w529, "Max Velocity to Home"=w527, "Mdrive Mode"=w528, "Device Name"="P") -> ("Moved"=→"MovedP":bool, "error out"=w531:errorcluster)  [unwired: 12 in, 1 out]
          }
        }
        n183 = case shown="True" w509 {
          tunnel: [_ w525] -> w505
          tunnel: w503 -> [_ w523]
          tunnel: w502 -> [_ w522]
          tunnel: w501 -> [_ w521]
          tunnel: w500 -> [_ w520]
          frame False {
          }
          frame True {
            n184 = call "LP MDrive_Home.vi"("VISA IN"=w523, "Home Direction"=w522, "Max Velocity to Home"=w520, "Mdrive Mode"=w521, "Device Name"="R") -> ("Moved"=→"MovedR":bool, "error out"=w525:errorcluster)  [unwired: 12 in, 1 out]
          }
        }
        n185 = case shown="True" w508 {
          tunnel: [_ w518] -> w504
          tunnel: w503 -> [_ w516]
          tunnel: w502 -> [_ w515]
          tunnel: w501 -> [_ w514]
          tunnel: "7000" ("Max Velocity to Home") -> [_ w513]
          frame False {
          }
          frame True {
            n186 = call "LP MDrive_Home.vi"("VISA IN"=w516, "Home Direction"=w515, "Max Velocity to Home"=w513, "Mdrive Mode"=w514, "Device Name"="Y") -> ("Moved"=→"MovedY":bool, "error out"=w518:errorcluster)  [unwired: 12 in, 1 out]
          }
        }
        n187 = Merge Errors(w506, w505, w504) -> (w507:errorcluster)
      }
      frame "ErrorHandling" {
        n188 = Unbundle By Name(w535) -> ("code"=w534:i32)
        n189 = case shown="1" w534 {
          frame 0, Default {
          }
          frame 1 {
          }
        }
        "last error" <- w535
      }
      frame "CloseMotor" {
        n190 = Unbundle By Name(w539) -> ("VISA resource name"=w538:refnum<visa-resource-name>)
        n191 = call "MDrive_Close_Com.vi"("VISA resource name in"=w538) -> ()  [unwired: 3 in]
      }
    }
    "error out" <- w36
    "output cluster" <- w32
  }
  n192 = timed-loop {
    tunnel: w9 -> [_]
    timing: w3 -> [_]
    timing-out: [_] -> w2
    stop <- FALSE stop-if-true
    (unwired) Motor_Loop_Mode_Typedef."NotActive" ("MotorLoopMode")
    n193 = node-c288() -> ()  [unwired: 1 in, 1 out]
    n194 = local read "output cluster"() -> (w542:T3)
    n195 = Unbundle By Name(w542) -> ("VISA resource name"=w547:refnum<visa-resource-name>, "Pactive"=w546:bool, "Ractive"=w545:bool, "Yactive"=w544:bool)
    n196 = global read "LP Globals.vi" "MotorLoopMode"() -> (w543:T2)
    "MotorLoopMode" <- w543
    n197 = Equal?(x=Motor_Loop_Mode_Typedef."Closed Loop", y=w543) -> (x = y?=w548:bool)
    n198 = case shown="\"Closed Loop\", \"ClosedOnce\"" w543 {
      selector: w543 -> [_ _ w597]
      tunnel: w547 -> [_ w576 w617]
      tunnel: w548 -> [_ _ _]
      tunnel: w546 -> [_ w582 w622]
      tunnel: w545 -> [_ w578 w619]
      tunnel: w544 -> [_ w577 w618]
      tunnel: w542 -> [_ _ w613]
      tunnel: [u32 1000 ("millisecond multiple") u32 200 ("millisecond multiple") u32 200 ("millisecond multiple")] -> w541
      frame "NotActive", Default {
      }
      frame "Open Loop" {
        n199 = Tick Count (ms)() -> (millisecond timer value=w581:u32)
        n200 = feedback-in #2(w581) -> ()
        n201 = feedback #2() -> (w580:u32)  [unwired: 1 in]
        n202 = Subtract(x=w581, y=w580) -> (x-y=→"open Loope Cycle Time":u32)
        n203 = global read "LP Globals.vi" "YawRatio"() -> (w558:i32)
        n204 = call "Check Position and Moving flag.vi"("Device Name"="P", "Axis Active"=w582, "VISA Refnum in"=w576) -> ("error out"=w570:errorcluster, "MovingFlag"=w583:bool, "Numeric"=w565:i32)  [unwired: 6 in]
        n205 = call "Check Position and Moving flag.vi"("Device Name"="R", "Axis Active"=w578, "VISA Refnum in"=w576) -> ("error out"=w569:errorcluster, "MovingFlag"=w573:bool, "Numeric"=w566:i32)  [unwired: 6 in]
        n206 = call "Check Position and Moving flag.vi"("Device Name"="Y", "Axis Active"=w577, "VISA Refnum in"=w576) -> ("error out"=w568:errorcluster, "MovingFlag"=w572:bool, "Numeric"=w557:i32)  [unwired: 6 in]
        n207 = Divide(x=w557, y=w558) -> (x/y=w556:dbl)
        n208 = Subtract(x=w565, y=w566) -> (x-y=w561:i32)
        n209 = Merge Errors(w570, w569, w568) -> (w567:errorcluster)
        n210 = Add(x=w565, y=w566) -> (x+y=w564:i32)
        n211 = Divide(x=w564, y=2) -> (x/y=w562:dbl)
        n212 = Bundle(w562, w561, w556, "MovingFlag"=w583, "MovingFlag"=w573, "MovingFlag"=w572) -> (w571:T19)  [unwired: 1 in]
        "MotPosition" <- w571
        n213 = local write "RT Loop Error"(w567) -> ()
        n214 = global write "LP Globals.vi" "MotPosition"(w571) -> ()
      }
      frame "Closed Loop", "ClosedOnce" {
        n215 = global read "LP Globals.vi" "Velocity"() -> (w600:i32)
        "Velocity" <- w600
        n216 = global read "LP Globals.vi" "Roll Gain"() -> (w599:i32)
        "Roll Gain" <- w599
        n217 = global read "LP Globals.vi" "Pitch Gain"() -> (w598:i32)
        "Pitch Gain" <- w598
        n218 = global read "LP Globals.vi" "Yaw Gain"() -> (w584:i32)
        n219 = Tick Count (ms)() -> (millisecond timer value=w621:u32)
        n220 = feedback-in #3(w621) -> ()
        n221 = feedback #3() -> (w620:u32)  [unwired: 1 in]
        n222 = Subtract(x=w621, y=w620) -> (x-y=→"Closed Loope Cycle Time":u32)
        n223 = global read "LP Globals.vi" "YawRatio"() -> (w586:i32)
        n224 = call "Check Position and Moving flag.vi"("Device Name"="P", "Axis Active"=w622, "VISA Refnum in"=w617) -> ("error out"=w610:errorcluster, "MovingFlag"=w623:bool, "Numeric"=w602:i32)  [unwired: 6 in]
        n225 = call "Check Position and Moving flag.vi"("Device Name"="R", "Axis Active"=w619, "VISA Refnum in"=w617) -> ("error out"=w608:errorcluster, "MovingFlag"=w616:bool, "Numeric"=w601:i32)  [unwired: 6 in]
        n226 = call "Check Position and Moving flag.vi"("Device Name"="Y", "Axis Active"=w618, "VISA Refnum in"=w617) -> ("error out"=w612:errorcluster, "MovingFlag"=w615:bool, "Numeric"=w587:i32)  [unwired: 6 in]
        n227 = call "LP Set Slew Speed for 3 axis.vi"("Max Speed"=w600, "Yaw Gain"=w584, "Pitch Gain"=w598, "Roll Gain"=w599, "output cluster"=w613) -> ("error out"=w609:errorcluster, "InRange"=w596:bool)  [unwired: 5 in]
        n228 = Divide(x=w587, y=w586) -> (x/y=w585:dbl)
        n229 = Add(x=w601, y=w602) -> (x+y=w604:i32)
        n230 = Subtract(x=w602, y=w601) -> (x-y=w590:i32)
        n231 = Divide(x=w604, y=2) -> (x/y=w591:dbl)
        n232 = Bundle(w591, w590, w585, "MovingFlag"=w623, "MovingFlag"=w616, "MovingFlag"=w615) -> (w614:T19)  [unwired: 1 in]
        n233 = Merge Errors(w609, w610, w608, w612) -> (→"RT Loop Error":errorcluster)
        n234 = global write "LP Globals.vi" "MotPosition"(w614) -> ()
        n235 = local write "MotPosition"(w614) -> ()
        n236 = call "LP Check Motors limits.vi"("RollPos"=w590, "PitchPos"=w591) -> ()  [unwired: 8 in, 2 out]
        n237 = case shown="\"ClosedOnce\"" w597 {
          tunnel: w596 -> [_ w625]
          frame "NotActive", Default {
          }
          frame "ClosedOnce" {
            n238 = case shown="False" w625 {
              frame False {
              }
              frame True {
                n239 = global read "LP Globals.vi" "Motor Loop Q"() -> (w627:refnum<queue>)
                n240 = global write "LP Globals.vi" "MotorLoopMode"(Motor_Loop_Mode_Typedef."Open Loop" ("MotorLoopMode")) -> ()
                n241 = call "LP Send Cmd Done.vi"("CMD"="DoLevel") -> ()  [unwired: 11 in]
                n242 = Enqueue Element(queue=w627, element=T8 {"CMD"=enum."StopMotion", "Data"=variant}) -> ()  [unwired: 2 in, 3 out]
              }
            }
          }
        }
        n243 = global read "LP Globals.vi" "EngageMotors"() -> (w594:bool)
        n244 = global read "LP Globals.vi" "EMGC Stop"() -> (w595:bool)
        n245 = Not(x=w594) -> (.not. x?=w593:bool)
        n246 = Or(x=w593, y=w595) -> (x .or. y?=w592:bool)
        n247 = case shown="True" w592 {
          frame False {
          }
          frame True {
            n248 = global write "LP Globals.vi" "MotorLoopMode"(Motor_Loop_Mode_Typedef."Open Loop" ("MotorLoopMode")) -> ()
          }
        }
      }
    }
    n249 = node-c288(w541) -> ()  [unwired: 1 out]
  }
  n250 = node-c288(w2) -> ()  [unwired: 1 out]
